vi "Wrist Tuner.vi"() -> ()   [LabVIEW 2018]
uses:
  <vilib>/Rock Robotics/WPI/ThirdParty/Phoenix-LabVIEW/Motor Controller/Controls/CTRE_Phoenix_MotorControl_ControlMode.ctl
  Support Code/Wrist Angle.vi
  <vilib>/Rock Robotics/WPI/ThirdParty/Phoenix-LabVIEW/Motor Controller/Get/CTRE_Phoenix_MotorController_GetSelectedSensorData.vi
  <vilib>/Rock Robotics/WPI/ThirdParty/Phoenix-LabVIEW/Motor Controller/Get/CTRE_Phoenix_MotorController_GetClosedLoopData.vi
  <vilib>/Rock Robotics/WPI/ThirdParty/Phoenix-LabVIEW/Motor Controller/Get/CTRE_Phoenix_MotorController_GetOutputCurrent_Enhanced.vi
panel:
  in  "Open Loop Override":bool
  in  "90* holding value":dbl=0.08
  in  "Enable OL FF":bool=TRUE
  in  "Open Loop":dbl(slide)=-1.1102230246251565e-16 scale=-1.0..1.0
  in  "Zero":bool
  out "Integral Accumulator":dbl=-9224.0
  out "Closed-loop Error":i32=3
  out "Velocity (Raw Sensor Units per 100 ms)":i32=840
  in  "Max Velocity":dbl=3000.0
  in  "Max Accel":dbl=3000.0
  in  "PID Constants":T1={"P Gain"=1.0, "I Gain"=0.004, "D Gain"=0.2, "F Gain"=0.0, "I Zone"=200.0, "Min Output"=-1.0, "Max Output"=1.0}
  in  "Setpoint":dbl
  out "Output Current":dbl
  out "Waveform Chart":T2(graph)={"Setpoint"=0.0, "Position (Raw Sensor Units)"=-3, "Velocity (Raw Sensor Units per 100 ms)"=0}
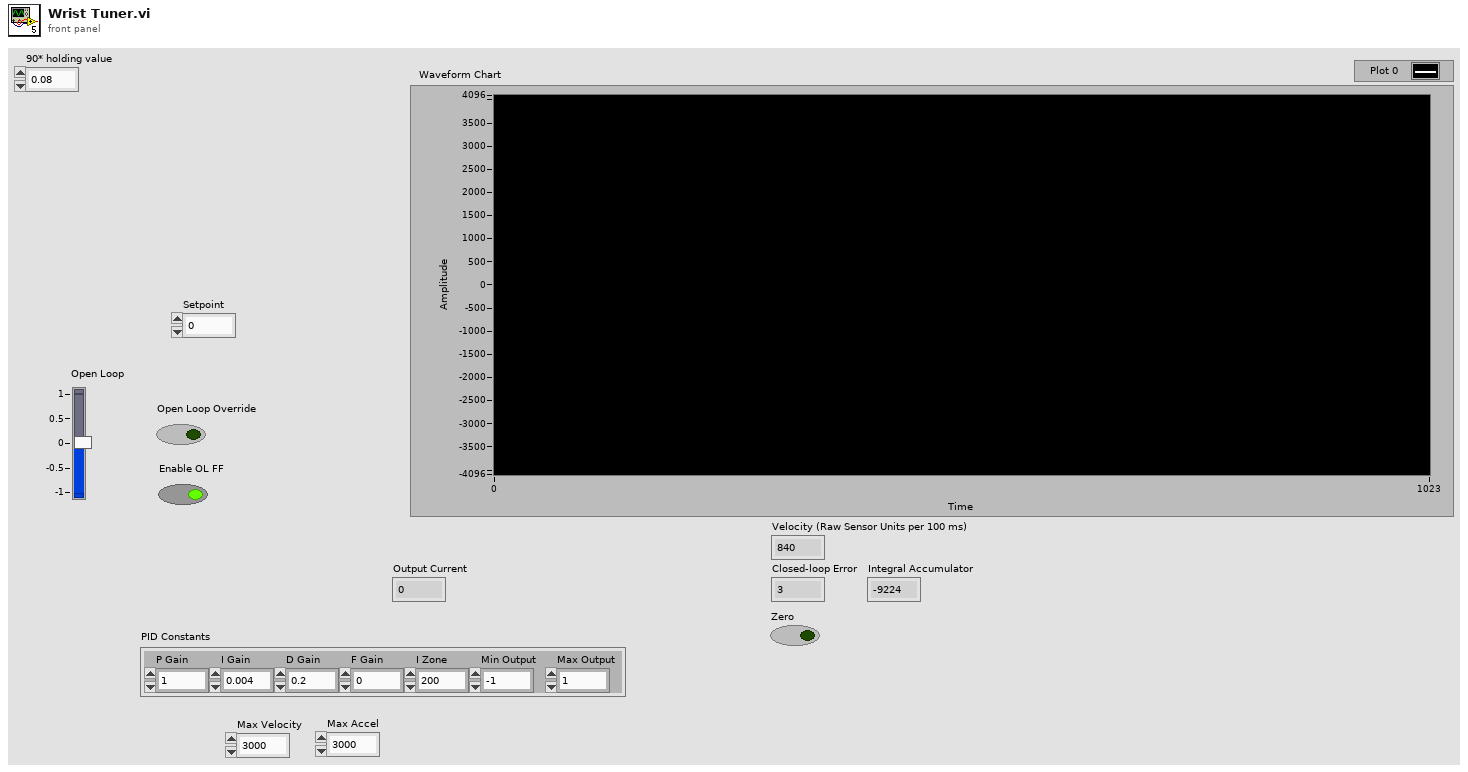
[diagram p1: front panel]
types:
  T1 = cluster{"P Gain":dbl, "I Gain":dbl, "D Gain":dbl, "F Gain":dbl, "I Zone":dbl, "Min Output":dbl, "Max Output":dbl}
  T2 = cluster{"Setpoint":dbl, "Position (Raw Sensor Units)":i32, "Velocity (Raw Sensor Units per 100 ms)":i32}
  T3 = typedef "WPI_MotorControlDeviceRef.ctl" = cluster{"DeviceStatus":errorcluster, "Type":T4, "PWM":cluster{"PWM Channel":T5, "DeadBand":T6}, "CAN":cluster{"Device Number":u8, "SetOutput VI Ref":variant, "GetOutput VI Ref":variant, "Enable VI Ref":variant, "Disable VI Ref":variant, "Data":variant}, "Invert":bool, "DIO PWM":cluster{"PWM \"Enable\" Channel":T5, "DIOChannel":T7, "PWM Rate":dbl}}
  T4 = typedef "WPI_MotorControlType.ctl" = enum16{"PWM", "CAN", "DIO PWM"}
  T5 = typedef "FPGA_DIOPWMChannel.ctl" = enum8{"PWM 0", "PWM 1", "PWM 2", "PWM 3", "PWM 4", "PWM 5", "PWM 6", "PWM 7", "PWM 8", "PWM 9", "PWM MXP 0", "PWM MXP 1", "PWM MXP 2", "PWM MXP 3", "PWM MXP 4", "PWM MXP 5", "PWM MXP 6", "PWM MXP 7", "PWM MXP 8", "PWM MXP 9", "Invalid"}
  T6 = typedef "WPI_PWMDeadband.ctl" = cluster{"Name":string, "maxPositivePwm":i32, "minPositivePwm":i32, "centerPwm":i32, "maxNegativePwm":i32, "minNegativePwm":i32, "angularRange":u16}
  T7 = typedef "FPGA_DIOChannel.ctl" = enum8{"DIO 0", "DIO 1", "DIO 2", "DIO 3", "DIO 4", "DIO 5", "DIO 6", "DIO 7", "DIO 8", "DIO 9", "DIO MXP 0", "DIO MXP 1", "DIO MXP 2", "DIO MXP 3", "DIO MXP 4", "DIO MXP 5", "DIO MXP 6", "DIO MXP 7", "DIO MXP 8", "DIO MXP 9", "DIO MXP 10", "DIO MXP 11", "DIO MXP 12", "DIO MXP 13", "DIO MXP 14", "DIO MXP 15", "SPI Port CS1", "SPI Port CS2", "SPI Port CS3", "SPI Port MISO", "SPI Port MOSI", "Invalid"}
  T8 = cluster{"P Gain":bool, "I Gain":bool, "D Gain":bool, "F Gain":bool, "I Zone":bool, "Min Output":bool, "Max Output":bool}
  T9 = enum16{"DemandType_Neutral", "DemandType_AuxPID", "DemandType_ArbitraryFeedForward"}
  T10 = typedef "CTRE_Phoenix_MotorControl_ControlMode.ctl" = u16
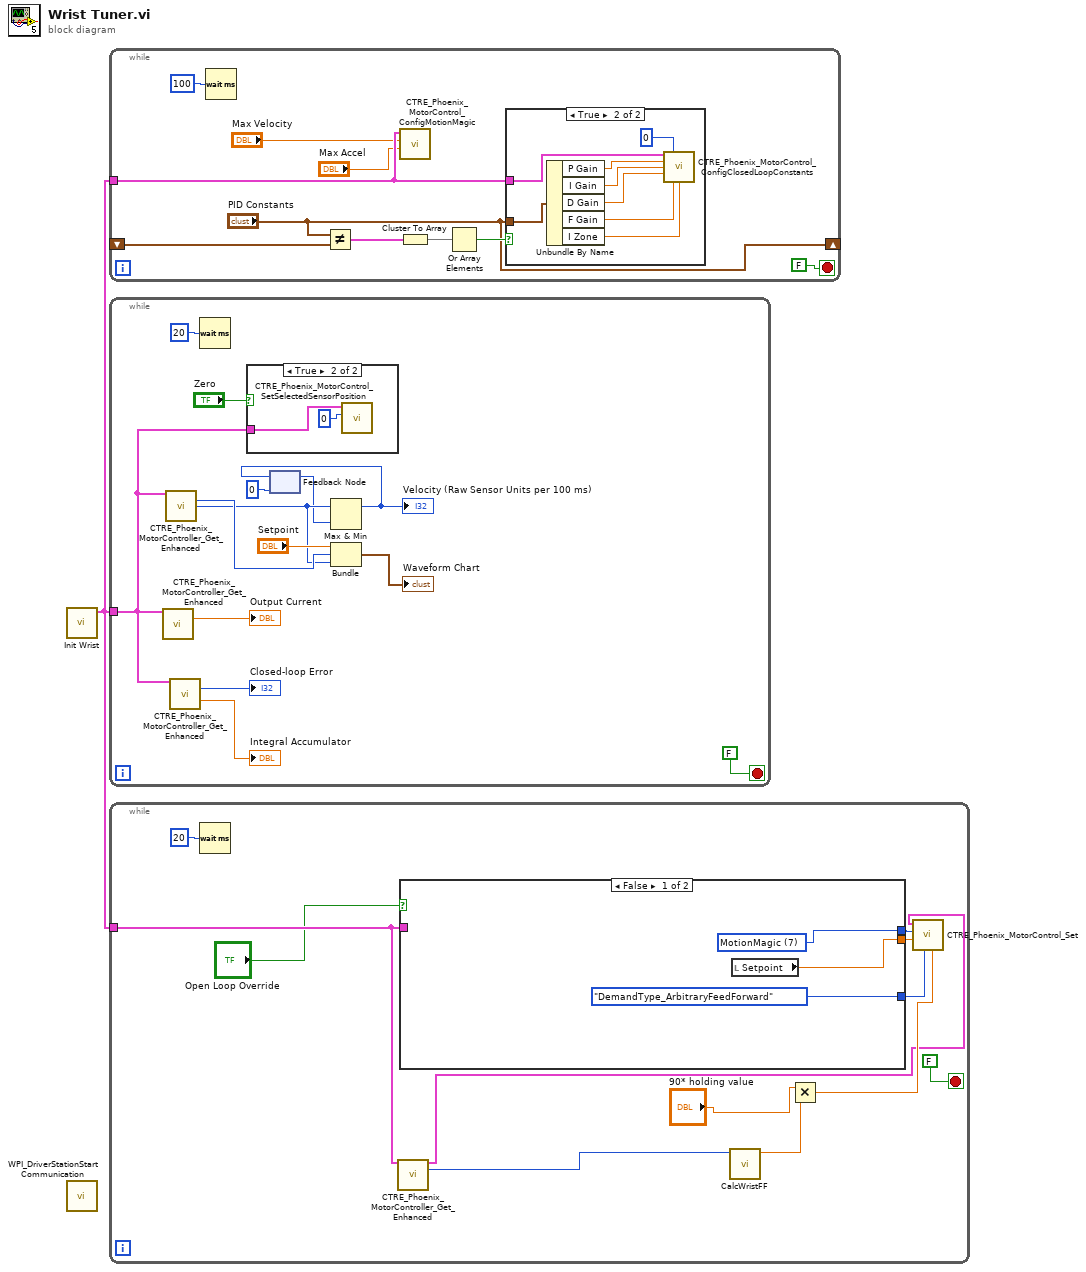
[diagram p0: block diagram]
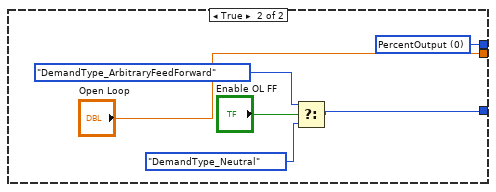
[diagram p2: hidden frame]
diagram:
  n1 = call "Init Wrist.vi"() -> ("Wrist Out"=w1:T3)  [unwired: 11 in]
  n2 = call <vilib>:"WPI_DriverStationStart Communication.vi"() -> ()  [unwired: 12 in]
  n3 = while {
    shift-right: ["PID Constants"] -> _
    shift-left: _ -> [w11]
    tunnel: w1 -> [w4]
    stop <- FALSE stop-if-true
    n4 = Wait (ms)(milliseconds to wait=u32 100) -> ()  [unwired: 1 out]
    n5 = Not Equal?(x="PID Constants", y=w11) -> (x != y?=w10:T8)
    n6 = call <vilib>:"CTRE_Phoenix_MotorControl_ConfigMotionMagic.vi"("Acceleration"="Max Accel", "Cruise Velocity"="Max Velocity", "PhoenixMotorControlDevRef"=w4) -> ()  [unwired: 7 in, 2 out]
    n7 = Cluster To Array(cluster=w10) -> (array=w9:bool[])
    n8 = Or Array Elements(Boolean array=w9) -> (logical OR=w8:bool)
    n9 = case shown="True" w8 {
      tunnel: w4 -> [_ w19]
      tunnel: "PID Constants" -> [_ w18]
      frame False {
      }
      frame True {
        n10 = Unbundle By Name(w18) -> ("P Gain"=w17:dbl, "I Gain"=w16:dbl, "D Gain"=w15:dbl, "F Gain"=w12:dbl, "I Zone"=w14:dbl)
        n11 = call <vilib>:"CTRE_Phoenix_MotorControl_ConfigClosedLoopConstants.vi"("PhoenixMotorControlDevRef"=w19, "slotIdx"=0, "P"=w17, "I"=w16, "D"=w15, "F"=w12, "I Zone"=w14) -> ()  [unwired: 7 in, 2 out]
      }
    }
  }
  n12 = while {
    tunnel: w1 -> [w20]
    stop <- FALSE stop-if-true
    n13 = call-poly <vilib>:"CTRE_Phoenix_MotorController_Get_Enhanced.vi"("PhoenixMotorControlDevRef"=w20) -> ("Output Current"=→"Output Current":dbl)  [unwired: 12 in, 2 out]
    n14 = call-poly <vilib>:"CTRE_Phoenix_MotorController_Get_Enhanced.vi"("PhoenixMotorControlDevRef"=w20) -> ("Position (Raw Sensor Units)"=w30:i32, "Velocity (Raw Sensor Units per 100 ms)"=w27:i32)  [unwired: 11 in, 2 out]
    n15 = call-poly <vilib>:"CTRE_Phoenix_MotorController_Get_Enhanced.vi"("PhoenixMotorControlDevRef"=w20) -> ("Closed-loop Error"=→"Closed-loop Error":i32, "Integral Accumulator"=→"Integral Accumulator":dbl)  [unwired: 9 in, 4 out]
    n16 = Wait (ms)(milliseconds to wait=u32 20) -> ()  [unwired: 1 out]
    n17 = case shown="True" "Zero" {
      tunnel: w20 -> [_ w34]
      frame False {
      }
      frame True {
        n18 = call <vilib>:"CTRE_Phoenix_MotorControl_SetSelectedSensorPosition.vi"("New Sensor Position"=0, "PhoenixMotorControlDevRef"=w34) -> ()  [unwired: 8 in, 2 out]
      }
    }
    n19 = feedback #1(0) -> (w26:i32)
    n20 = Max & Min(x=w27, y=w26) -> (max(x,y)=w25:i32)  [unwired: 1 out]
    "Velocity (Raw Sensor Units per 100 ms)" <- w25
    n21 = feedback-in #1(w25) -> ()
    n22 = Bundle("Setpoint"="Setpoint", "Position (Raw Sensor Units)"=w30, "Velocity (Raw Sensor Units per 100 ms)"=w27) -> (→"Waveform Chart":T2)  [unwired: 1 in]
  }
  n23 = while {
    tunnel: w1 -> [w40]
    stop <- FALSE stop-if-true
    n24 = Wait (ms)(milliseconds to wait=u32 20) -> ()  [unwired: 1 out]
    n25 = call-poly <vilib>:"CTRE_Phoenix_MotorController_Get_Enhanced.vi"("PhoenixMotorControlDevRef"=w40) -> ("PhoenixMotorControlDevRef"=w39:T3, "Position (Raw Sensor Units)"=w37:i32)  [unwired: 11 in, 2 out]
    n26 = case shown="False" "Open Loop Override" {
      tunnel: w40 -> [_ _]
      tunnel: [T9."DemandType_ArbitraryFeedForward" ("DemandType") w51] -> w43
      tunnel: [w49 "Open Loop"] -> w42
      tunnel: [w48 w54] -> w41
      frame False {
        w48 = T10 7 items=["PercentOutput"=0, "Position"=1, "Velocity"=2, "Current"=3, "Follower"=5, "MotionProfile"=6, "MotionMagic"=7, "MotionProfileArc"=10, "Disabled"=15] ("Control Mode")
        n27 = local read "Setpoint"() -> (w49:dbl)
      }
      frame True {
        w54 = T10 0 items=["PercentOutput"=0, "Position"=1, "Velocity"=2, "Current"=3, "Follower"=5, "MotionProfile"=6, "MotionMagic"=7, "MotionProfileArc"=10, "Disabled"=15] ("Control Mode")
        n28 = Select(t=T9."DemandType_ArbitraryFeedForward" ("DemandType"), s="Enable OL FF", f=T9."DemandType_Neutral" ("DemandType")) -> (s? t:f=w51:T9)
      }
    }
    n29 = call "CalcWristFF.vi"("Ticks (from vertical)"=w37) -> ("Vert Force Scalar"=w38:dbl)  [unwired: 10 in]
    n30 = Multiply(x="90* holding value", y=w38) -> (x*y=w44:dbl)
    n31 = call <vilib>:"CTRE_Phoenix_MotorControl_Set.vi"("Demand1"=w44, "DemandType"=w43, "Output"=w42, "Control Mode"=w41, "PhoenixMotorControlDevRef"=w39) -> ()  [unwired: 5 in, 2 out]
  }
